vi "Host - Mode Colour change.vi"(9 "Text Color":u32(colorbox), 10 "BG Color":u32(colorbox), 11 "TabControl in":refnum<vi>) -> ()   [LabVIEW 2021]
panel:
  out "Array":string[](array[string])
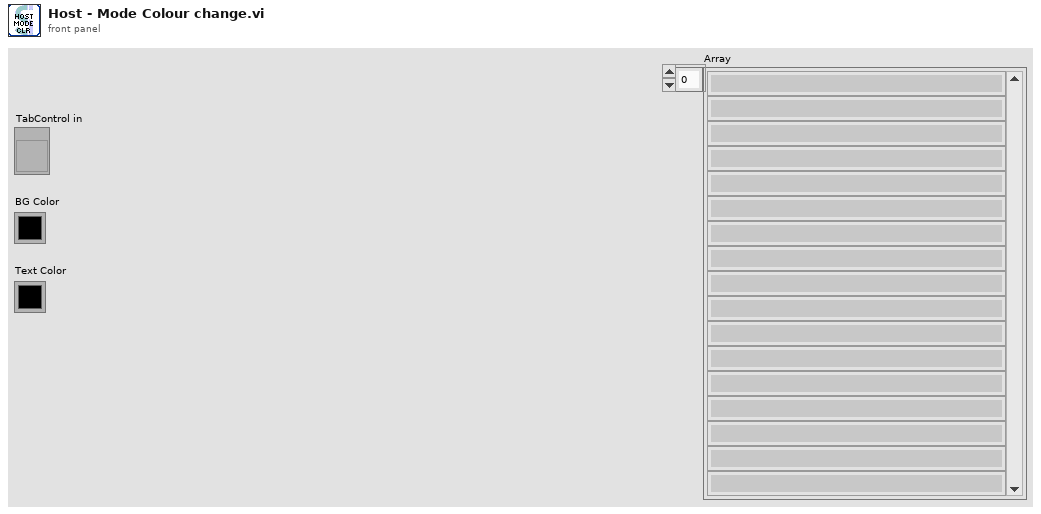
[diagram p1: front panel]
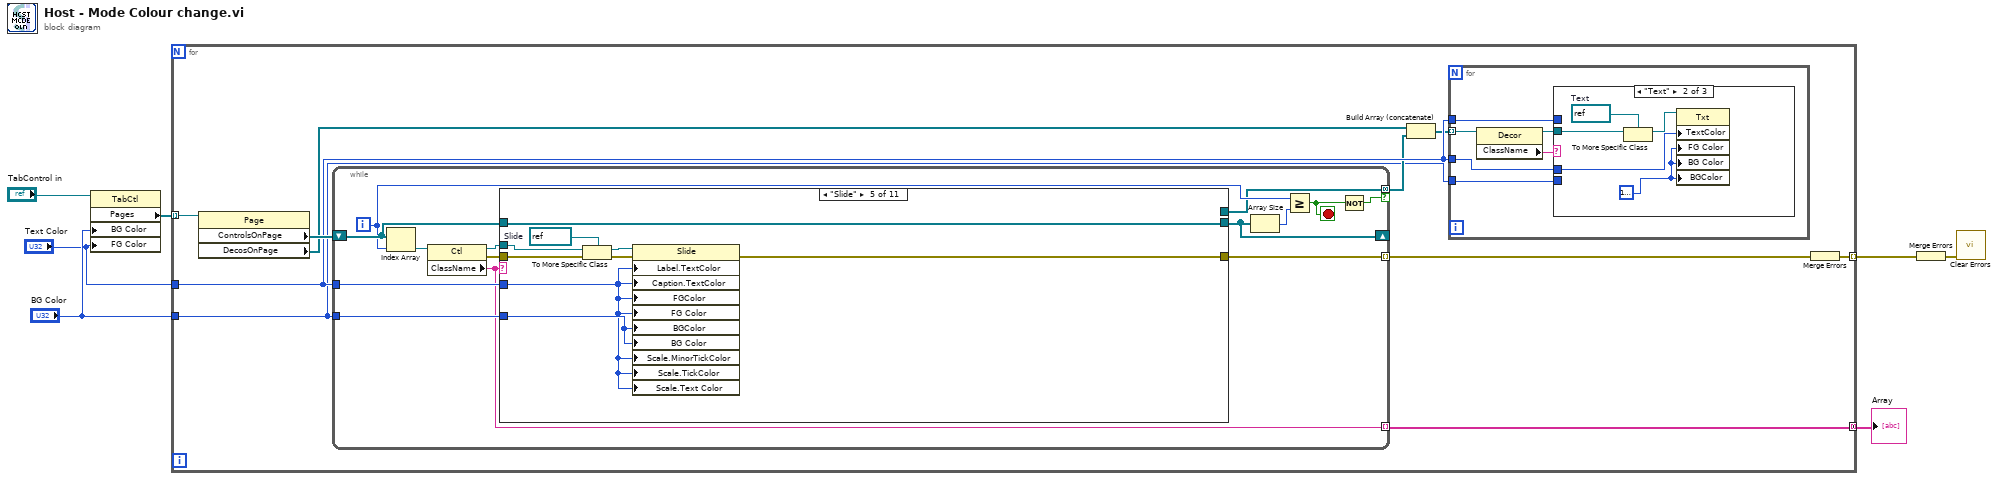
[diagram p0: block diagram]
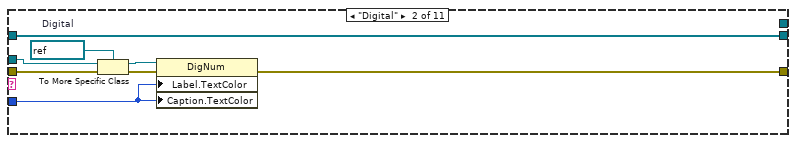
[diagram p3: hidden frame]
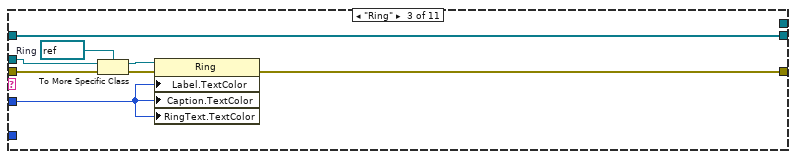
[diagram p4: hidden frame]
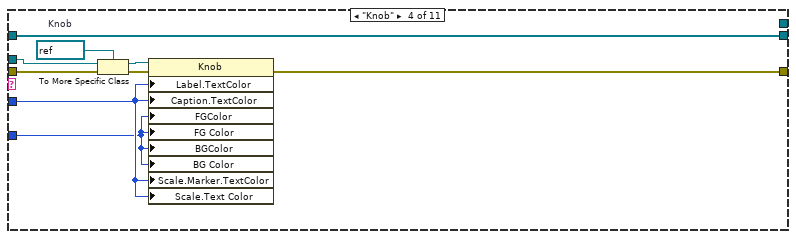
[diagram p5: hidden frame]
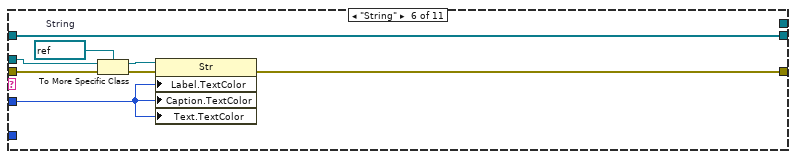
[diagram p6: hidden frame]
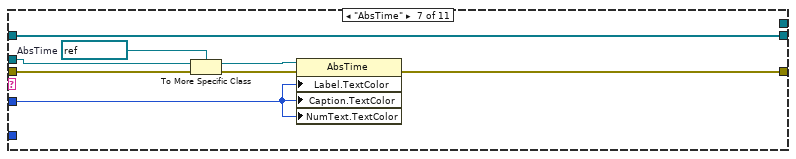
[diagram p7: hidden frame]
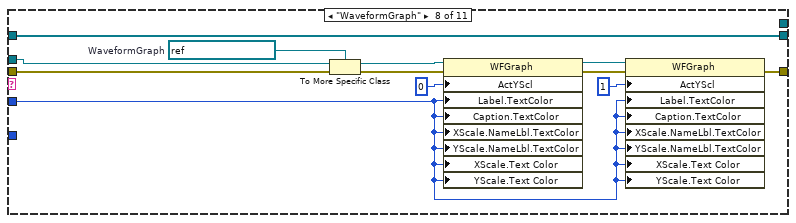
[diagram p8: hidden frame]
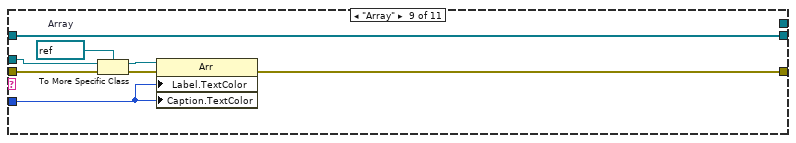
[diagram p9: hidden frame]
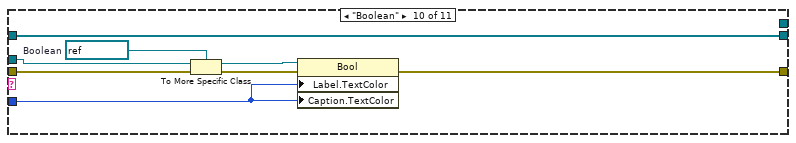
[diagram p10: hidden frame]
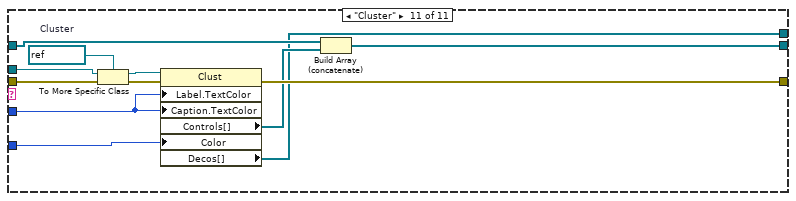
[diagram p11: hidden frame]
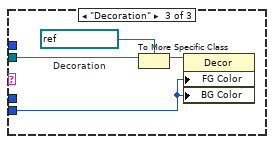
[diagram p13: hidden frame]
diagram:
  n1 = property class="TabCtl"(reference="TabControl in", "BG Color"="BG Color", "FG Color"="Text Color") -> ("Pages"=w7:refnum<vi>[])  [unwired: 1 in, 2 out]
  n2 = for {
    tunnel: w7 -> [w17] mode=indexing
    tunnel: "Text Color" -> [w13]
    tunnel: [w12] -> w5 mode=indexing
    tunnel: "BG Color" -> [w8]
    tunnel: [w9] -> w3 mode=concatenating
    n3 = property class="Page"(reference=w17) -> ("ControlsOnPage"=w16:refnum<vi>[], "DecosOnPage"=w14:refnum<vi>[])  [unwired: 1 in, 2 out]
    n4 = while {
      tunnel: w13 -> [w30]
      tunnel: [w29] -> w15 mode=indexing
      shift-right: [w26] -> _
      shift-left: w16 -> [w27]
      tunnel: w8 -> [w22]
      tunnel: [w21] -> w10 mode=concatenating if=w19
      tunnel: [w18] -> w9 mode=indexing
      i -> [w24]
      stop <- w20 stop-if-true
      n5 = Index Array(array=w27, index=w24) -> (element=w28:refnum<vi>)
      n6 = property class="Ctl"(reference=w28) -> (reference out=w31:refnum<vi>, error out=w23:errorcluster, "ClassName"=w18:string)  [unwired: 1 in]
      n7 = case shown="\"Slide\"" w18 {
        tunnel: w31 -> [_ w41 w49 w58 w67 w75 w83 w95 w103 w111 w123]
        tunnel: w30 -> [_ w34 w46 w51 w59 w72 w80 w91 w100 w108 w120]
        tunnel: [w32 w38 w45 w55 w64 w71 w78 w87 w99 w107 w119] -> w29
        tunnel: w27 -> [w33 w37 w44 w54 w63 w70 w77 w85 w98 w106 w118]
        tunnel: [w33 w37 w44 w54 w63 w70 w77 w85 w98 w106 w116] -> w26
        tunnel: w23 -> [w32 w36 w42 w52 w61 w69 w76 w84 w97 w104 w115]
        tunnel: w22 -> [_ _ _ w50 w60 _ _ _ _ _ w113]
        tunnel: [_ _ _ _ _ _ _ _ _ _ w112] -> w21
        frame Default {
        }
        frame "Digital" {
          w40 = refnum<vi> refnum  # Digital
          n8 = To More Specific Class(target class=w40, reference=w41, error in=w36) -> (specific class reference=w39:refnum<vi>, error out=w35:errorcluster)
          n9 = property class="DigNum"(reference=w39, error in=w35, "Label.TextColor"=w34, "Caption.TextColor"=w34) -> (error out=w38:errorcluster)  [unwired: 1 out]
        }
        frame "Ring" {
          w48 = refnum<vi> refnum  # Ring
          n10 = To More Specific Class(target class=w48, reference=w49, error in=w42) -> (specific class reference=w47:refnum<vi>, error out=w43:errorcluster)
          n11 = property class="Ring"(reference=w47, error in=w43, "Label.TextColor"=w46, "Caption.TextColor"=w46, "RingText.TextColor"=w46) -> (error out=w45:errorcluster)  [unwired: 1 out]
        }
        frame "Knob" {
          w57 = refnum<vi> refnum  # Knob
          n12 = To More Specific Class(target class=w57, reference=w58, error in=w52) -> (specific class reference=w56:refnum<vi>, error out=w53:errorcluster)
          n13 = property class="Knob"(reference=w56, error in=w53, "Label.TextColor"=w51, "Caption.TextColor"=w51, "FGColor"=w50, "FG Color"=w50, "BGColor"=w50, "BG Color"=w50, "Scale.Marker.TextColor"=w51, "Scale.Text Color"=w51) -> (error out=w55:errorcluster)  [unwired: 1 out]
        }
        frame "Slide" {
          w66 = refnum<vi> refnum  # Slide
          n14 = To More Specific Class(target class=w66, reference=w67, error in=w61) -> (specific class reference=w65:refnum<vi>, error out=w62:errorcluster)
          n15 = property class="Slide"(reference=w65, error in=w62, "Label.TextColor"=w59, "Caption.TextColor"=w59, "FGColor"=w59, "FG Color"=w59, "BGColor"=w60, "BG Color"=w60, "Scale.MinorTickColor"=w59, "Scale.TickColor"=w59, "Scale.Text Color"=w59) -> (error out=w64:errorcluster)  [unwired: 1 out]
        }
        frame "String" {
          w74 = refnum<vi> refnum  # String
          n16 = To More Specific Class(target class=w74, reference=w75, error in=w69) -> (specific class reference=w73:refnum<vi>, error out=w68:errorcluster)
          n17 = property class="Str"(reference=w73, error in=w68, "Label.TextColor"=w72, "Caption.TextColor"=w72, "Text.TextColor"=w72) -> (error out=w71:errorcluster)  [unwired: 1 out]
        }
        frame "AbsTime" {
          w82 = refnum<vi> refnum  # AbsTime
          n18 = To More Specific Class(target class=w82, reference=w83, error in=w76) -> (specific class reference=w81:refnum<vi>, error out=w79:errorcluster)
          n19 = property class="AbsTime"(reference=w81, error in=w79, "Label.TextColor"=w80, "Caption.TextColor"=w80, "NumText.TextColor"=w80) -> (error out=w78:errorcluster)  [unwired: 1 out]
        }
        frame "WaveformGraph" {
          w94 = refnum<vi> refnum  # WaveformGraph
          n20 = To More Specific Class(target class=w94, reference=w95, error in=w84) -> (specific class reference=w93:refnum<vi>, error out=w92:errorcluster)
          n21 = property class="WFGraph"(reference=w93, error in=w92, "ActYScl"=u32 0 ("Active Plot"), "Label.TextColor"=w91, "Caption.TextColor"=w91, "XScale.NameLbl.TextColor"=w91, "YScale.NameLbl.TextColor"=w91, "XScale.Text Color"=w91, "YScale.Text Color"=w91) -> (reference out=w88:refnum<vi>, error out=w86:errorcluster)
          n22 = property class="WFGraph"(reference=w88, error in=w86, "ActYScl"=u32 1 ("Active Plot"), "Label.TextColor"=w91, "Caption.TextColor"=w91, "XScale.NameLbl.TextColor"=w91, "YScale.NameLbl.TextColor"=w91, "XScale.Text Color"=w91, "YScale.Text Color"=w91) -> (error out=w87:errorcluster)  [unwired: 1 out]
        }
        frame "Array" {
          w102 = refnum<vi> refnum  # Array
          n23 = To More Specific Class(target class=w102, reference=w103, error in=w97) -> (specific class reference=w101:refnum<vi>, error out=w96:errorcluster)
          n24 = property class="Arr"(reference=w101, error in=w96, "Label.TextColor"=w100, "Caption.TextColor"=w100) -> (error out=w99:errorcluster)  [unwired: 1 out]
        }
        frame "Boolean" {
          w110 = refnum<vi> refnum  # Boolean
          n25 = To More Specific Class(target class=w110, reference=w111, error in=w104) -> (specific class reference=w109:refnum<vi>, error out=w105:errorcluster)
          n26 = property class="Bool"(reference=w109, error in=w105, "Label.TextColor"=w108, "Caption.TextColor"=w108) -> (error out=w107:errorcluster)  [unwired: 1 out]
        }
        frame "Cluster" {
          w122 = refnum<vi> refnum  # Cluster
          n27 = To More Specific Class(target class=w122, reference=w123, error in=w115) -> (specific class reference=w121:refnum<vi>, error out=w114:errorcluster)
          n28 = property class="Clust"(reference=w121, error in=w114, "Label.TextColor"=w120, "Caption.TextColor"=w120, "Color"=w113) -> (error out=w119:errorcluster, "Controls[]"=w117:refnum<vi>[], "Decos[]"=w112:refnum<vi>[])  [unwired: 1 out]
          n29 = Build Array (concatenate)(w118, w117) -> (w116:refnum<vi>[])
        }
      }
      n30 = Array Size(array=w26) -> (size(s)=w25:i32)
      n31 = Greater Or Equal?(x=w24, y=w25) -> (x >= y?=w20:bool)
      n32 = Not(x=w20) -> (.not. x?=w19:bool)
    }
    n33 = Build Array (concatenate)(w14, w10) -> (w11:refnum<vi>[])
    n34 = for {
      tunnel: w11 -> [w129] mode=indexing
      tunnel: w13 -> [w127]
      tunnel: w8 -> [w126]
      tunnel: w13 -> [w124]
      n35 = property class="Decor"(reference=w129) -> (reference out=w125:refnum<vi>, "ClassName"=w128:string)  [unwired: 1 in, 1 out]
      n36 = case shown="\"Text\"" w128 {
        tunnel: w127 -> [_ w132 _]
        tunnel: w126 -> [_ _ w135]
        tunnel: w125 -> [_ w131 w136]
        tunnel: w124 -> [_ _ _]
        frame "False", Default {
        }
        frame "Text" {
          w130 = u32 16777216
          w134 = refnum<vi> refnum  # Text
          n37 = To More Specific Class(target class=w134, reference=w131) -> (specific class reference=w133:refnum<vi>)  [unwired: 1 in, 1 out]
          n38 = property class="Txt"(reference=w133, "TextColor"=w132, "FG Color"=w130, "BG Color"=w130, "BGColor"=w130) -> ()  [unwired: 1 in, 2 out]
        }
        frame "Decoration" {
          w138 = refnum<vi> refnum  # Decoration
          n39 = To More Specific Class(target class=w138, reference=w136) -> (specific class reference=w137:refnum<vi>)  [unwired: 1 in, 1 out]
          n40 = property class="Decor"(reference=w137, "FG Color"=w135, "BG Color"=w135) -> ()  [unwired: 1 in, 2 out]
        }
      }
    }
    n41 = Merge Errors(w15) -> (w12:errorcluster)
  }
  "Array" <- w3
  n42 = Merge Errors(w5) -> (w4:errorcluster)
  n43 = call <vilib>:"Clear Errors.vi"("error in (no error)"=w4) -> ()  [unwired: 5 in, 2 out]
